vi "action.vi"(0 "HGF_Device_SelfTest":refnum<class "HGF_Device_SelfTest.lvclass">, 2 "HGF_Visitable":refnum<class "HGF_Visitable.lvclass">, 5 "error in (no error)":errorcluster) -> (14 "dup HGF_Device_SelfTest":refnum<class "HGF_Device_SelfTest.lvclass">, 16 "dup HGF_Visitable":refnum<class "HGF_Visitable.lvclass">, 19 "error out":errorcluster)   [LabVIEW 2014, in "HGF_DeviceBaseClasses.lvlib" / "HGF_Device_SelfTest.lvclass"]
doc: "This is a dynamic dispatch VI that is called from Visitor.visit(). It will call member VIs of Visitable to perform the requested action which means: calling public methods of Visitable child class.\n\n<B>Hint:</B> This method is abstract and need to be implemented by child classes."
uses:
  HGF_Device_SelfTest.lvclass
  HGF_DeviceBase/HGF_DeviceBase.lvclass
  HGF_BaseClasses/HGF_Visitable/HGF_Visitable.lvclass
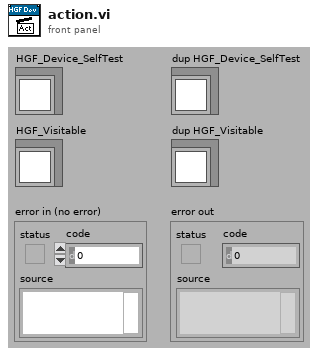
[diagram p1: front panel]
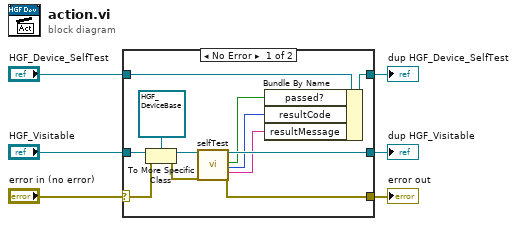
[diagram p0: block diagram]
diagram:
  n1 = case shown="No Error" "error in (no error)" {
    selector: "error in (no error)" -> [w16 w20]
    tunnel: "HGF_Visitable" -> [w18 w21]
    tunnel: [w14 w21] -> w5
    tunnel: [w12 w20] -> w3
    tunnel: [w10 w19] -> w1
    tunnel: "HGF_Device_SelfTest" -> [w11 w19]
    frame No Error {
      n2 = To More Specific Class(target class=refnum<class "HGF_DeviceBase.lvclass"> refnum ("HGF_DeviceBaseClasses.lvlib:HGF_DeviceBase.lvclass"), reference=w18, error in=w16) -> (specific class reference=w15:refnum<class "HGF_DeviceBase.lvclass">, error out=w13:errorcluster)
      n3 = call-dynamic "selfTest.vi"("HGF_DeviceBase"=w15, "error in (no error)"=w13) -> ("dup HGF_DeviceBase"=w14:refnum<class "HGF_DeviceBase.lvclass">, "passed?"=w9:bool, "resultCode"=w8:i32, "resultMessage"=w7:string, "error out"=w12:errorcluster)  [unwired: 13 out]
      n4 = Bundle By Name(cluster=w11, "passed?"=w9, "resultCode"=w8, "resultMessage"=w7) -> (w10:refnum<class "HGF_Device_SelfTest.lvclass">)
    }
    frame Error {
    }
  }
  "error out" <- w3
  "dup HGF_Device_SelfTest" <- w1
  "dup HGF_Visitable" <- w5
